vi "makeResult.vi"(8 "error in (no error)":errorcluster, 11 "TextTestRunner in":refnum<class "TextTestRunner.JUnitXML.lvclass">) -> (0 "error out":errorcluster, 2 "TestResult":refnum<class "TestResult.lvclass">, 3 "TextTestRunner out":refnum<class "TextTestRunner.JUnitXML.lvclass">)   [LabVIEW 2011, in "TextTestRunner.JUnitXML.lvclass"]
uses:
  TextTestRunner.JUnitXML.lvclass
  <vilib>/addons/_JKI Toolkits/VI Tester/TestResult.llb/TestResult.lvclass
  _TextTestResult.Ant/_TextTestResult.JUnitXML.lvclass
  <vilib>/addons/_JKI Toolkits/VI Tester/_TextTestResult.llb/_TextTestResult.lvclass
  <vilib>/addons/_JKI Toolkits/VI Tester/TextTestRunner.llb/TextTestRunner.lvclass
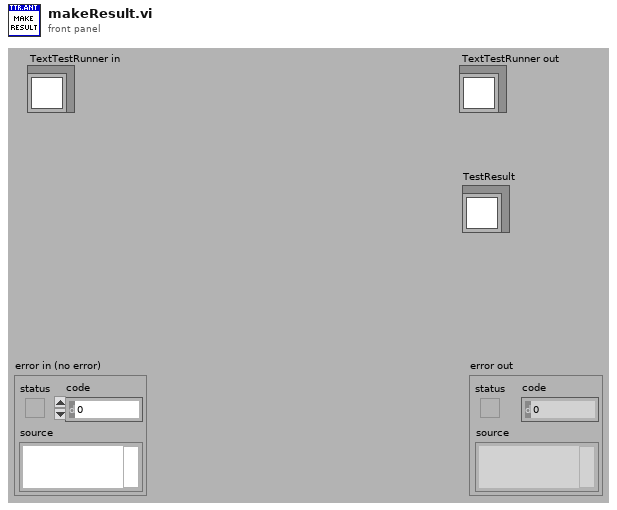
[diagram p1: front panel]
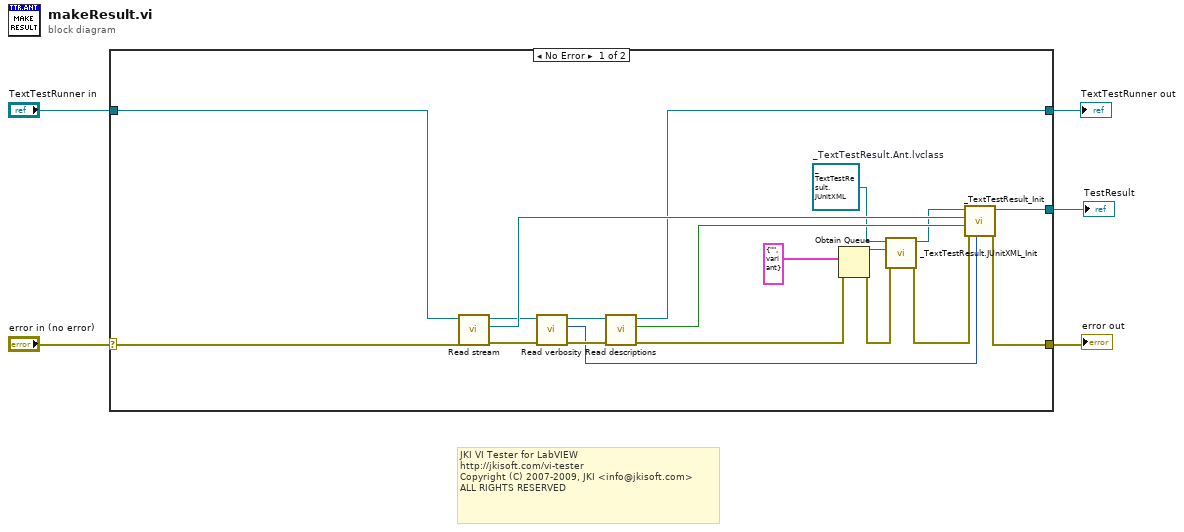
[diagram p0: block diagram]
diagram:
  # "JKI VI Tester for LabVIEW\nhttp://jkisoft.com/vi-tester\nCopyright (C) 2007-2009, JKI <info@jkisoft.com>\nALL RIGHTS RESERVED"
  n1 = case shown="No Error" "error in (no error)" {
    selector: "error in (no error)" -> [w11 w26]
    tunnel: [w24 w26] -> w4
    tunnel: [w12 w25] -> w2
    tunnel: "TextTestRunner in" -> [w10 w25]
    tunnel: [w23 _] -> w1
    frame No Error {
      w15 = refnum<class "_TextTestResult.JUnitXML.lvclass"> refnum  # _TextTestResult.Ant.lvclass
      n2 = call <vilib>:"Read stream.vi"("error in (no error)"=w11, "TextTestRunner in"=w10) -> ("error out"=w21:errorcluster, "stream"=w22:refnum<queue>, "TextTestRunner out"=w18:refnum<class "TextTestRunner.JUnitXML.lvclass">)  [unwired: 7 in]
      n3 = call <vilib>:"Read verbosity.vi"("error in (no error)"=w21, "TextTestRunner in"=w18) -> ("error out"=w20:errorcluster, "verbosity"=w16:u32, "TextTestRunner out"=w19:refnum<class "TextTestRunner.JUnitXML.lvclass">)  [unwired: 7 in]
      n4 = call <vilib>:"Read descriptions.vi"("error in (no error)"=w20, "TextTestRunner in"=w19) -> ("error out"=w7:errorcluster, "descriptions"=w17:bool, "TextTestRunner out"=w12:refnum<class "TextTestRunner.JUnitXML.lvclass">)  [unwired: 7 in]
      n5 = Obtain Queue(element data type=cluster{"Type":string, "Data":variant} {"Type"="", "Data"=variant} ("element"), error in (no error)=w7) -> (queue out=w8:refnum<queue>, error out=w6:errorcluster)  [unwired: 3 in, 1 out]
      n6 = call "_TextTestResult.JUnitXML_Init.vi"("error in (no error)"=w6, "stream.Results"=w8, "TestTestResult in"=w15) -> ("error out"=w13:errorcluster, "TestTestResult out"=w14:refnum<class "_TextTestResult.JUnitXML.lvclass">)  [unwired: 7 in]
      n7 = call <vilib>:"_TextTestResult_Init.vi"("verbosity"=w16, "error in (no error)"=w13, "descriptions"=w17, "stream"=w22, "TestTestResult in"=w14) -> ("error out"=w24:errorcluster, "TestTestResult out"=w23:refnum<class "_TextTestResult.JUnitXML.lvclass">)  [unwired: 5 in]
    }
    frame Error {
    }
  }
  "error out" <- w4
  "TextTestRunner out" <- w2
  "TestResult" <- w1
